vi "Sequencer Do.vi"(8 "error in (no error)":errorcluster, 10 "Sequencer in":refnum<class "Sequencer.lvclass">, 11 "Nested Sequence Msg":refnum<class "Nested Sequence Msg.lvclass">) -> (0 "error out":errorcluster, 2 "Sequencer out":refnum<class "Sequencer.lvclass">)   [LabVIEW 2020, in "Sequencer.lvlib" / "Nested Sequence Msg.lvclass"]
doc: "Do nothing."
uses:
  Nested Sequence Msg.lvclass
  Sequencer/Sequencer.lvclass
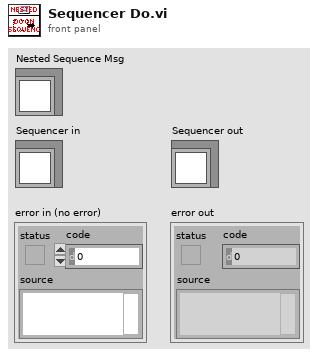
[diagram p1: front panel]
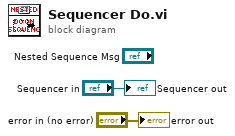
[diagram p0: block diagram]
diagram:
  "error out" <- "error in (no error)"
  "Sequencer out" <- "Sequencer in"
